vi "test_gauss.vi"() -> ()   [LabVIEW 2018]
uses:
  Control 1.ctl
  <vilib>/DAQmx/write.llb/DAQmx Write (Analog 1D Wfm NChan NSamp).vi
  <vilib>/Analysis/1siggen.llb/General Gauss-Mod Sine.vi
  <vilib>/DAQmx/create/channels.llb/DAQmx Create Channel (AO-Voltage-Basic).vi
  <vilib>/DAQmx/configure/timing.llb/DAQmx Timing (Sample Clock).vi
  <vilib>/DAQmx/miscellaneous.llb/DAQmx Fill In Error Info.vi
  <vilib>/Analysis/NI_AALBase.lvlib
  <resource>/objmgr/daqmx.rc
  <vilib>/measure/NI_MABase.lvlib
panel:
  in  "Chirp amplitude":dbl=1.0 format="%0.2f"
  in  "Gauss amplitude":dbl=1.0
  in  "delay":dbl
  in  "width":dbl=0.5
  in  "Sampling rate":dbl=799999.9999999999
  in  "f2":dbl=300.0 format="%0.2f"
  in  "f1":dbl=100.0 format="%0.2f"
  in  "Boolean":bool
  in  "Exit":bool
  out "Actual Sample Rate 2":dbl=800000.0 format="%0.2f"
  in  "Physical Channel(s)":tag="Dev3/ao0:1"
  in  "Min Voltage 2":dbl=-10.0
  in  "Max Voltage 2":dbl=10.0
  in  "Sample Clock Source":tag="OnboardClock"
  in  "Sample Rate 2":dbl=800000.0 format="%#_6p"
  in  "Pulser Cycles":i32=10
  out "Sample per Channel AO":dbl=26666.0
  in  "Pulse generator":T2={"Waveform Type"=2, "Amplitude"=1.0, "Frequency"=300.0} {"Frequency" format="%0.2p"; "Amplitude" format="%0.2p"; "Waveform Type" items=["Sine Wave", "Triangle Wave", "Square Wave", "Sawtooth Wave"]}
  in  "Duty cycle %":dbl=50.0 format="%#.2f"
  in  "normalized bandwidth":dbl=0.5
  in  "attenuation (dB)":dbl=7.0
  out "Waveform Graph":waveform(dbl)[](graph)=[{"t0"=timestamp(0 s since 1904-01-01), "dt"=1.25e-06, "Y"=array[40000 elements]}, {"t0"=timestamp(0 s since 1904-01-01), "dt"=1.25e-06, "Y"=array[40000 elements]}, {"t0"=timestamp(0 s since 1904-01-01), "dt"=1.25e-06, "Y"=array[40000 elements]}]
  in  "center frequency (Hz)":dbl=200.0
  in  "delay (s)":dbl=0.025
  in  "samples":i32=40000
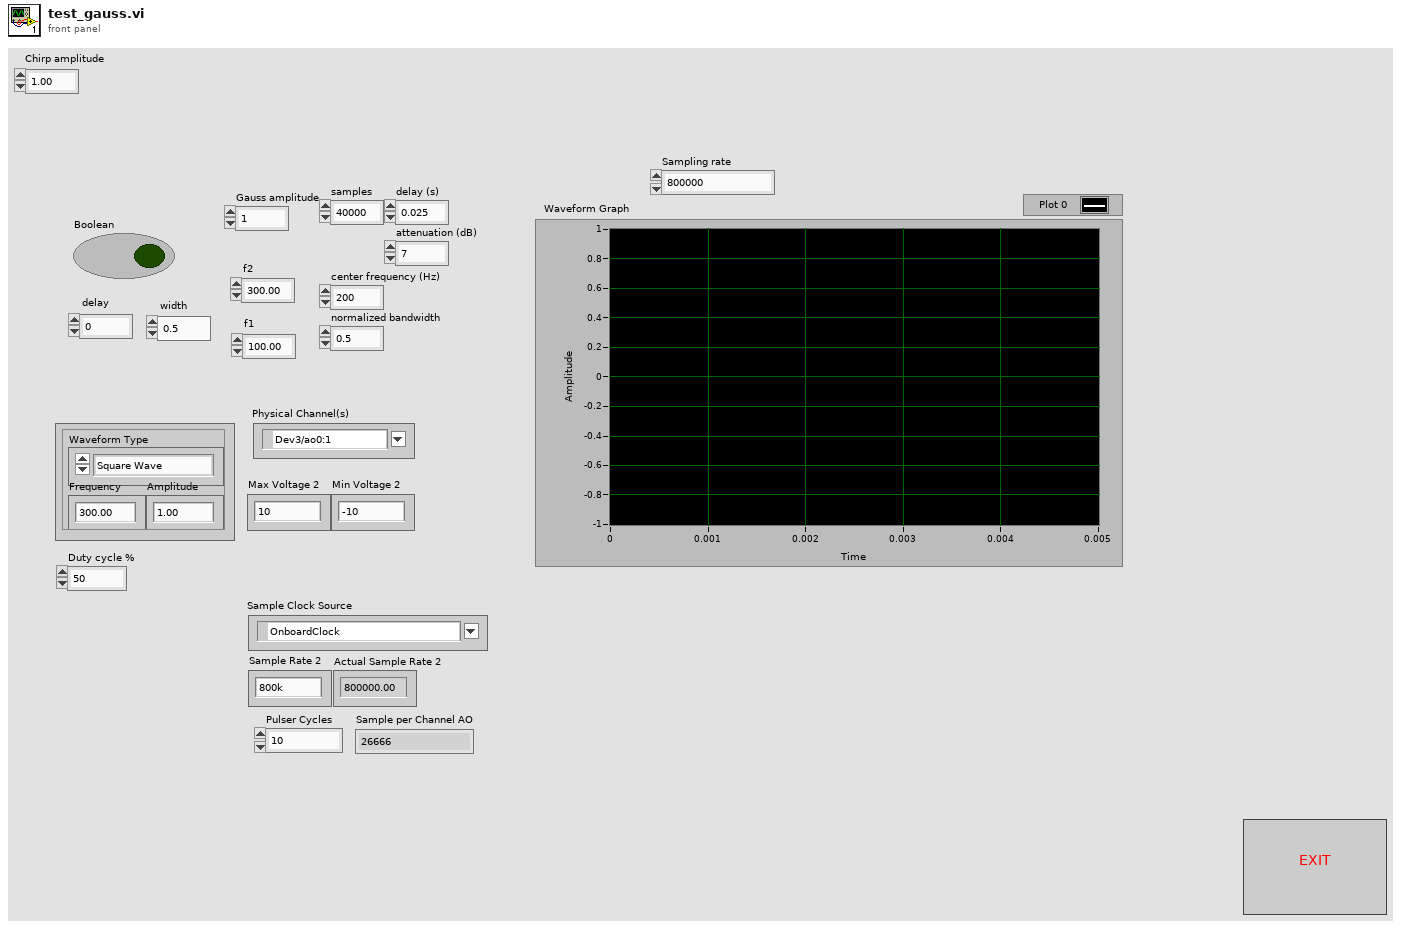
[diagram p1: front panel]
types:
  T1 = typedef "Control 1.ctl" = dbl
  T2 = cluster{"Waveform Type":u16, "Amplitude":T1, "Frequency":dbl}
  T3 = enum16{"Sine Wave", "Triangle Wave", "Square Wave", "Sawtooth Wave"}
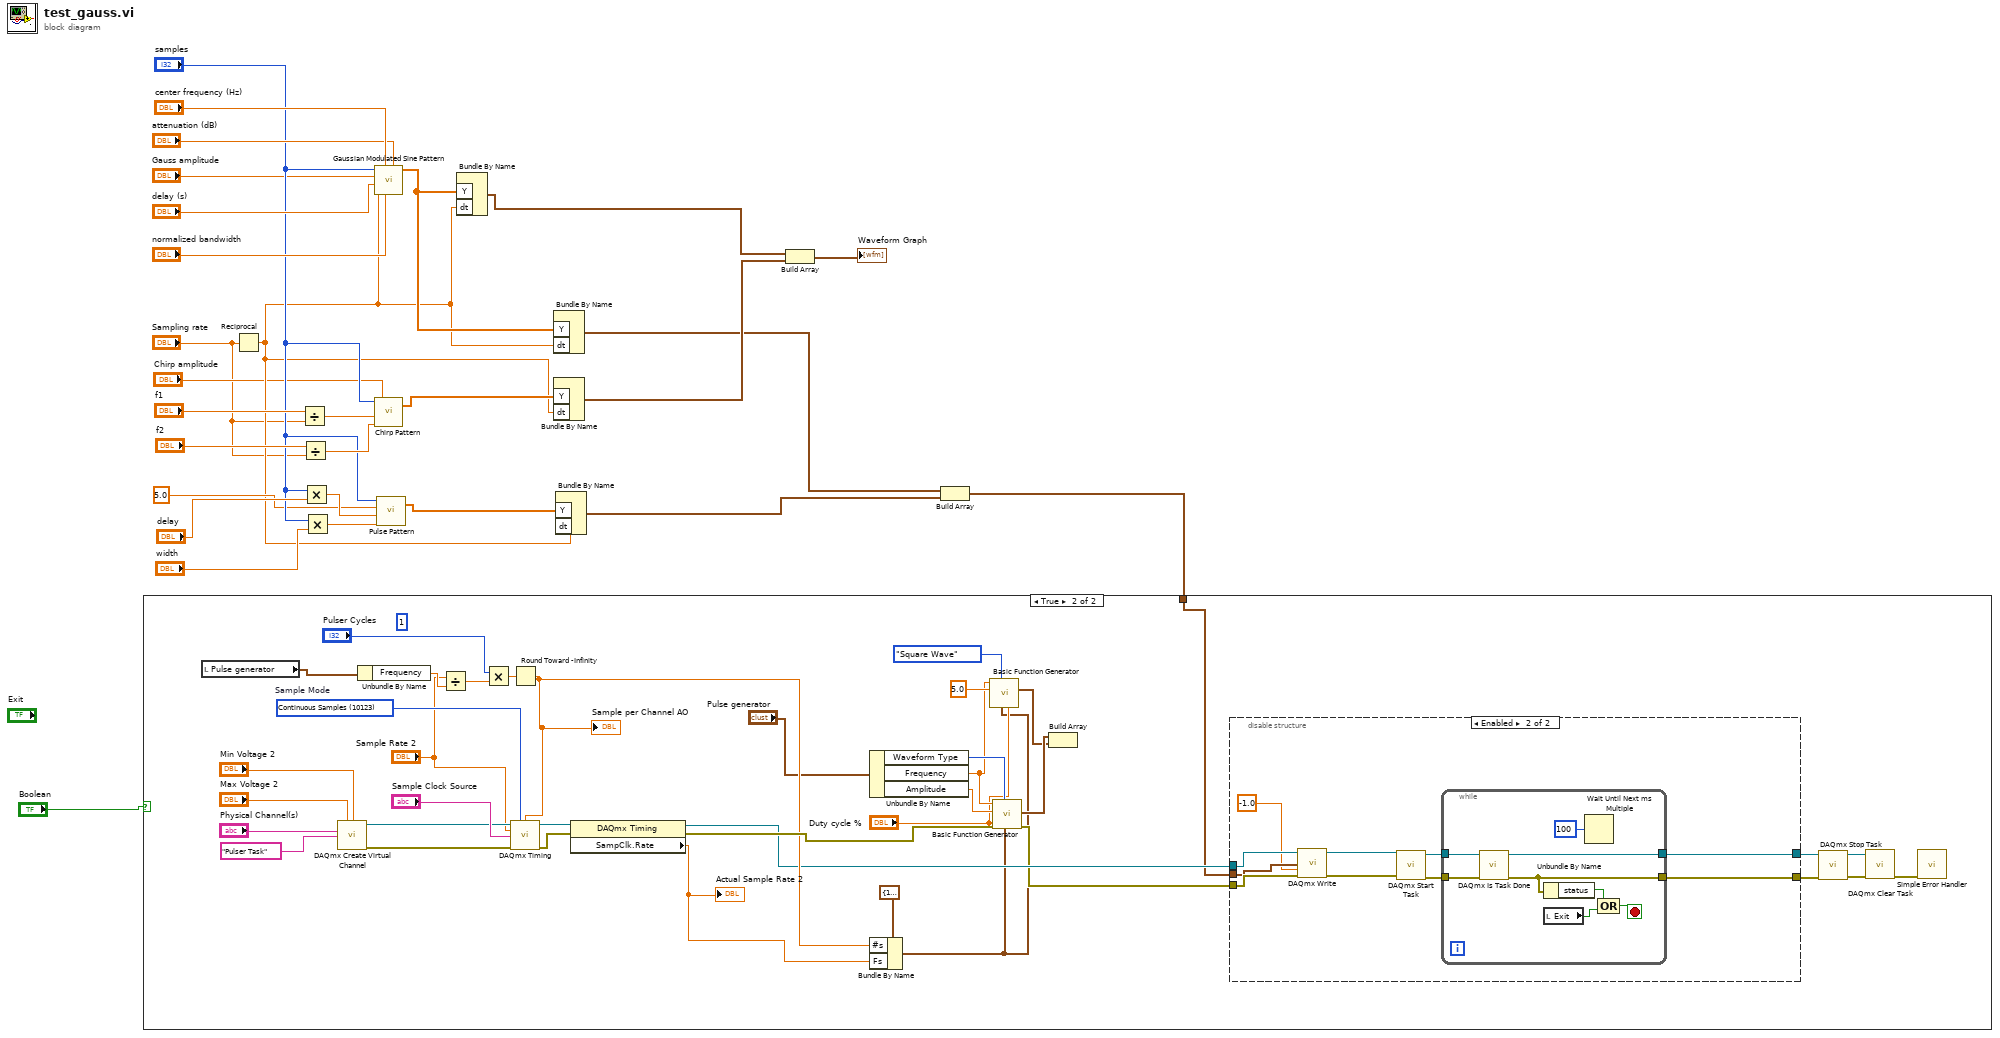
[diagram p0: block diagram]
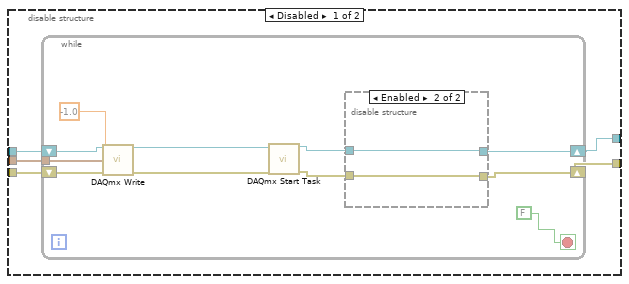
[diagram p3: hidden frame]
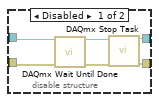
[diagram p4: hidden frame]
diagram:
  n1 = Reciprocal(x="Sampling rate") -> (1/x=w3:dbl)
  n2 = Divide(x="f1", y="Sampling rate") -> (x/y=w18:dbl)
  n3 = Divide(x="f2", y="Sampling rate") -> (x/y=w16:dbl)
  n4 = Multiply(x="samples", y="delay") -> (x*y=w10:dbl)
  n5 = Multiply(x="samples", y="width") -> (x*y=w11:dbl)
  n6 = call <vilib>:"Gaussian Modulated Sine Pattern.vi"("attenuation (dB)"="attenuation (dB)", "normalized bandwidth"="normalized bandwidth", "center frequency (Hz)"="center frequency (Hz)", "delta t (s)"=w3, "delay (s)"="delay (s)", "amplitude"="Gauss amplitude", "samples"="samples") -> ("Gauss-Mod Sine Pattern"=w24:dbl[])  [unwired: 3 in, 1 out]
  n7 = call <vilib>:"Chirp Pattern.vi"("f2"=w16, "f1"=w18, "amplitude"="Chirp amplitude", "samples"="samples") -> ("Chirp Pattern"=w20:dbl[])  [unwired: 1 out]
  n8 = call <vilib>:"Pulse Pattern.vi"("width"=w11, "delay"=w10, "amplitude"=5.0, "samples"="samples") -> ("Pulse Pattern"=w15:dbl[])  [unwired: 1 out]
  n9 = Bundle By Name("Y"=w24, "dt"=w3) -> (w22:waveform(dbl))  [unwired: 1 in]
  n10 = Bundle By Name("Y"=w24, "dt"=w3) -> (w4:waveform(dbl))  [unwired: 1 in]
  n11 = Bundle By Name("Y"=w20, "dt"=w3) -> (w5:waveform(dbl))  [unwired: 1 in]
  n12 = Bundle By Name("Y"=w15, "dt"=w3) -> (w8:waveform(dbl))  [unwired: 1 in]
  n13 = Build Array(w22, w5) -> (→"Waveform Graph":waveform(dbl)[])
  n14 = Build Array(w4, w8) -> (w7:waveform(dbl)[])
  n15 = case shown="True" "Boolean" {
    tunnel: w7 -> [_ w29]
    frame False {
    }
    frame True {
      (unwired) 1 ("x")
      w64 = 10123 items=["Finite Samples"=10178, "Continuous Samples"=10123, "Hardware Timed Single Point"=12522]  # Sample Mode
      n16 = local read "Pulse generator"() -> (w48:T2)
      n17 = call-poly <vilib>:"DAQmx Create Virtual Channel.vi"("maximum value"="Max Voltage 2", "minimum value"="Min Voltage 2", "physical channels"="Physical Channel(s)", "name to assign"="Pulser Task") -> ("task out"=w55:refnum<k21>, "error out"=w54:errorcluster)  [unwired: 10 in]
      n18 = Unbundle By Name(w48) -> ("Frequency"=w53:dbl)
      n19 = Divide(x="Sample Rate 2", y=w53) -> (x/y=w51:dbl)
      n20 = Multiply(x="Pulser Cycles", y=w51) -> (x*y=w50:dbl)
      n21 = Round Toward -Infinity(1:w50) -> (0:w49:dbl)
      "Sample per Channel AO" <- w49
      n22 = call-poly <vilib>:"DAQmx Timing.vi"("task/channels in"=w55, "sample mode"=w64, "samples per channel"=w49, "rate"="Sample Rate 2", "source"="Sample Clock Source", "error in"=w54) -> ("task out"=w66:refnum<k21>, "error out"=w65:errorcluster)  [unwired: 8 in]
      n23 = property class="DAQmx Timing"(reference=w66, error in=w65) -> (reference out=w47:refnum<k21>, error out=w58:errorcluster, "SampClk.Rate"=w56:dbl)
      "Actual Sample Rate 2" <- w56
      n24 = Unbundle By Name("Pulse generator") -> ("Waveform Type"=w45:u16, "Frequency"=w41:dbl, "Amplitude"=w44:T1)
      n25 = Bundle By Name(cluster=cluster{"Fs":dbl, "#s":dbl} {"Fs"=1000.0, "#s"=1000.0} ("sampling info"), "#s"=w49, "Fs"=w56) -> (w36:cluster{"Fs":dbl, "#s":dbl})
      n26 = call <vilib>:"Basic Function Generator.vi"("square wave duty cycle (%)"="Duty cycle %", "sampling info"=w36, "signal type"=T3."Square Wave", "amplitude"=5.0, "frequency"=w41) -> ("signal out"=w37:waveform(dbl))  [unwired: 4 in, 2 out]
      n27 = call <vilib>:"Basic Function Generator.vi"("square wave duty cycle (%)"="Duty cycle %", "sampling info"=w36, "signal type"=w45, "error in (no error)"=w58, "amplitude"=w44, "frequency"=w41) -> ("error out"=w46:errorcluster, "signal out"=w38:waveform(dbl))  [unwired: 3 in, 1 out]
      n28 = Build Array(w38, w37) -> ()  [unwired: 1 out]
      n29 = disable-structure shown="Enabled" {
        disable-tunnel: w29 -> [w71 w94]
        disable-tunnel: [w70 w93] -> w33
        disable-tunnel: [w69 w92] -> w30
        disable-tunnel: w47 -> [w68 w96]
        disable-tunnel: w46 -> [w67 w95]
        frame Disabled {
          n30 = while {
            tunnel: w71 -> [w82]
            shift-right: [w78] -> w70
            shift-left: w68 -> [w76]
            shift-right: [w77] -> w69
            shift-left: w67 -> [w75]
            stop <- FALSE stop-if-true
            n31 = call-poly <vilib>:"DAQmx Write.vi"("task/channels in"=w76, "data"=w82, "timeout"=-1.0, "error in"=w75) -> ("task out"=w81:refnum<k21>, "error out"=w80:errorcluster)  [unwired: 9 in, 1 out]
            n32 = call <vilib>:"DAQmx Start Task.vi"("task/channels in"=w81, "error in"=w80) -> ("task out"=w74:refnum<k21>, "error out"=w73:errorcluster)  [unwired: 12 in]
            n33 = disable-structure shown="Enabled" {
              disable-tunnel: [w88 w90] -> w78
              disable-tunnel: [w87 w89] -> w77
              disable-tunnel: w74 -> [w86 w90]
              disable-tunnel: w73 -> [w85 w89]
              frame Disabled {
                n34 = call <vilib>:"DAQmx Wait Until Done.vi"("task/channels in"=w86, "error in"=w85) -> ("task out"=w84:refnum<k21>, "error out"=w83:errorcluster)  [unwired: 12 in]
                n35 = call <vilib>:"DAQmx Stop Task.vi"("task/channels in"=w84, "error in"=w83) -> ("task out"=w88:refnum<k21>, "error out"=w87:errorcluster)  [unwired: 12 in]
              }
              frame Enabled {
              }
            }
          }
        }
        frame Enabled {
          n36 = call-poly <vilib>:"DAQmx Write.vi"("task/channels in"=w96, "data"=w94, "timeout"=-1.0, "error in"=w95) -> ("task out"=w98:refnum<k21>, "error out"=w100:errorcluster)  [unwired: 9 in, 1 out]
          n37 = call <vilib>:"DAQmx Start Task.vi"("task/channels in"=w98, "error in"=w100) -> ("task out"=w97:refnum<k21>, "error out"=w99:errorcluster)  [unwired: 12 in]
          n38 = while {
            tunnel: w97 -> [w108]
            tunnel: w99 -> [w107]
            tunnel: [w105] -> w92
            tunnel: [w106] -> w93
            stop <- w102 stop-if-true
            n39 = call <vilib>:"DAQmx Is Task Done.vi"("task/channels in"=w108, "error in"=w107) -> ("task out"=w106:refnum<k21>, "error out"=w105:errorcluster)  [unwired: 11 in, 1 out]
            n40 = Unbundle By Name(w105) -> ("status"=w103:bool)
            n41 = local read "Exit"() -> (w101:bool)
            n42 = Wait Until Next ms Multiple(millisecond multiple=u32 100) -> ()  [unwired: 1 out]
            n43 = Compound Arithmetic op=OR(w103, w101) -> (w102:bool)
          }
        }
      }
      n44 = call <vilib>:"DAQmx Stop Task.vi"("task/channels in"=w33, "error in"=w30) -> ("task out"=w32:refnum<k21>, "error out"=w31:errorcluster)  [unwired: 12 in]
      n45 = call <vilib>:"DAQmx Clear Task.vi"("task in"=w32, "error in"=w31) -> ("error out"=w63:errorcluster)  [unwired: 13 in]
      n46 = call <vilib>:"Simple Error Handler.vi"("error in (no error)"=w63) -> ()  [unwired: 4 in, 5 out]
    }
  }
